vi "command string.vi"(11 "DATA":u8[](array[numeric]) format="%02x") -> (3 "Command":string)   [LabVIEW 2013]
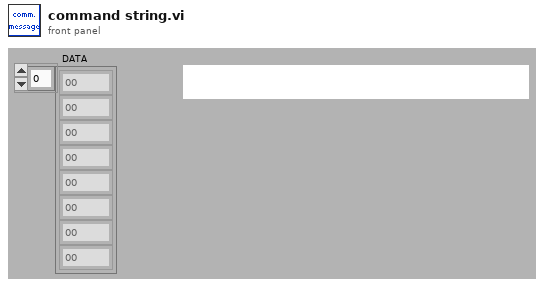
[diagram p1: front panel]
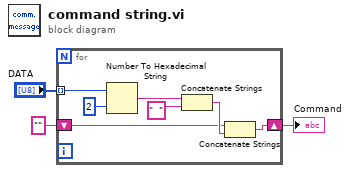
[diagram p0: block diagram]
diagram:
  n1 = for {
    tunnel: "DATA" -> [w9] mode=indexing
    shift-right: [w5] -> w1
    shift-left: "" -> [w4]
    n2 = Number To Hexadecimal String(1:i16 2 ("宽度(-)"), 2:w9) -> (0:w8:string)
    n3 = Concatenate Strings(w8, "  " ("字符串")) -> (w6:string)
    n4 = Concatenate Strings(w4, w6) -> (w5:string)
  }
  "Command" <- w1
